vi "GetLdNamesAndClasses.vi"(8 "error in (no error)":errorcluster caption="entrée d'erreur (pas d'erreur)", 11 "Experiment en entrée":refnum<class "Experiment.lvclass"> caption="DNL_LabVIEW Object in") -> (0 "error out":errorcluster caption="sortie d'erreur", 1 "LdClasses":string[](array[string]), 2 "LdNames":string[](array[string]), 3 "Experiment en sortie":refnum<class "Experiment.lvclass"> caption="DNL_LabVIEW Object out", 4 "LdNamesAndClasses":string[][](array[string]))   [LabVIEW 2019, in "Experiment.lvclass"]
uses:
  Experiment.lvclass
  Experiment.lvclass/Experiment.ctl
  DevicesClass/BaseDevice/BaseDevice.lvclass
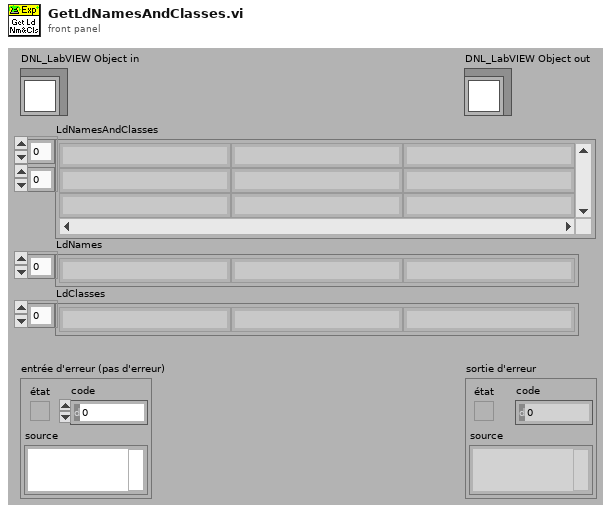
[diagram p1: front panel]
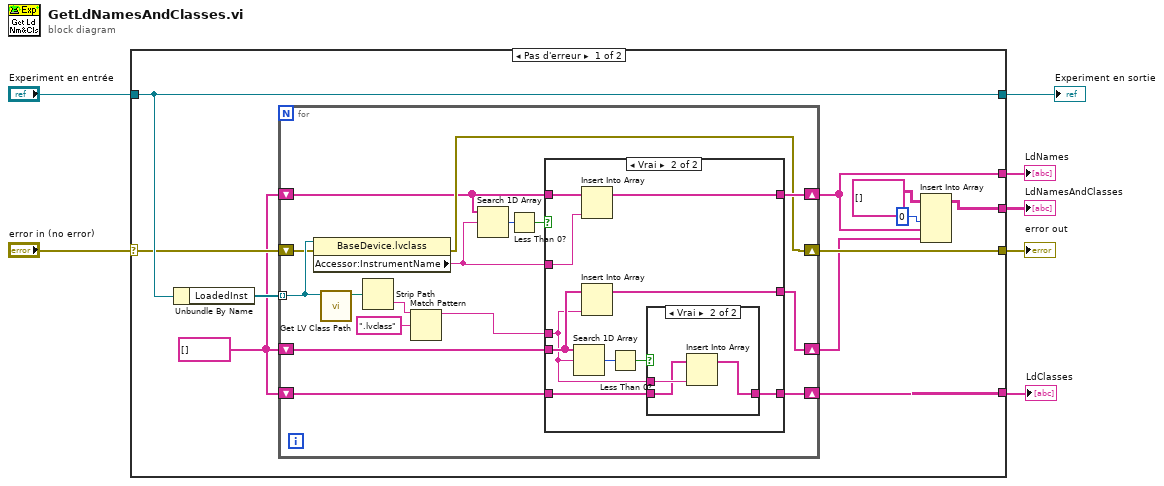
[diagram p0: block diagram]
diagram:
  n1 = case shown="Pas d'erreur" "error in (no error)" {
    selector: "error in (no error)" -> [w16 w53]
    tunnel: [w15 w53] -> w6
    tunnel: [w18 w52] -> w4
    tunnel: "Experiment en entrée" -> [w18 w52]
    tunnel: [w10 _] -> w3
    tunnel: [w11 _] -> w2
    tunnel: [w8 _] -> w1
    frame No Error {
      w9 = string[] []
      n2 = Unbundle By Name(w18) -> ("LoadedInst"=w17:refnum<class "BaseDevice.lvclass">[])
      n3 = for {
        tunnel: w17 -> [w31] mode=indexing
        shift-right: [w24] -> w15
        shift-left: w16 -> [w30]
        shift-right: [w26] -> w11
        shift-left: w9 -> [w23]
        shift-right: [w25] -> w12
        shift-left: w9 -> [w21]
        shift-right: [w20] -> w8
        shift-left: w9 -> [w19]
        n4 = property class="BaseDevice.lvclass"(reference=w31, error in=w30) -> (error out=w24:errorcluster, "Accessor:InstrumentName"=w22:string)  [unwired: 1 out]
        n5 = call <vilib>:"Get LV Class Path.vi"("object"=w31) -> ("class path"=w32:path)  [unwired: 9 in, 1 out]
        n6 = Strip Path(path=w32) -> (name=w34:string)  [unwired: 1 out]
        n7 = Match Pattern(string=w34, regular expression=".lvclass" ("expression régulière")) -> (before substring=w27:string)  [unwired: 1 in, 3 out]
        n8 = Search 1D Array(1D array=w23, element=w22) -> (index of element=w29:i32)  [unwired: 1 in]
        n9 = Less Than 0?(x=w29) -> (x < 0?=w28:bool)
        n10 = case shown="Vrai" w28 {
          tunnel: w27 -> [_ w38]
          tunnel: [w37 w46] -> w26
          tunnel: w23 -> [w37 w47]
          tunnel: [w35 w43] -> w25
          tunnel: w22 -> [_ w45]
          tunnel: w21 -> [w35 w42]
          tunnel: [w36 w40] -> w20
          tunnel: w19 -> [w36 w39]
          frame False {
            # "instrument name already in list"
          }
          frame True {
            n11 = Search 1D Array(1D array=w42, element=w38) -> (index of element=w44:i32)  [unwired: 1 in]
            n12 = Insert Into Array(array=w47, new element=w45) -> (w46:string[])  [unwired: 1 in]
            n13 = Insert Into Array(array=w42, new element=w38) -> (w43:string[])  [unwired: 1 in]
            n14 = Less Than 0?(x=w44) -> (x < 0?=w41:bool)
            n15 = case shown="Vrai" w41 {
              tunnel: [w48 w49] -> w40
              tunnel: w39 -> [w48 w50]
              tunnel: w38 -> [_ w51]
              frame False {
              }
              frame True {
                n16 = Insert Into Array(array=w50, new element=w51) -> (w49:string[])  [unwired: 1 in]
              }
            }
          }
        }
      }
      n17 = Insert Into Array(array=string[][] [] ("tableau ajouté"), index (col)=0 ("indice désactivé (col)"), new element #1=w11, new element #2=w12) -> (w10:string[][])  [unwired: 1 in]
    }
    frame Error {
    }
  }
  "error out" <- w6
  "Experiment en sortie" <- w4
  "LdNamesAndClasses" <- w3
  "LdNames" <- w2
  "LdClasses" <- w1
